vi "Get_Disc_Flow_Rate.vi"(9 "Jet Frequency":dbl, 10 "Radius":dbl[](array[numeric]), 11 "Phase Average":dbl[][](array[numeric])) -> (1 "time":dbl[](array[numeric]), 2 "|Qd|":dbl, 3 "Qd(t)":dbl[](array[numeric]))   [LabVIEW 2012]
uses:
  <vilib>/Analysis/2dsp.llb/Integral Method.ctl
  <vilib>/Analysis/1siggen.llb/Ramp Pattern by Samples.vi
  <vilib>/Analysis/8numeric.llb/1D Numeric Integration.vi
  <vilib>/Analysis/NI_AALBase.lvlib
  <vilib>/gmath/NI_Gmath.lvlib
  <vilib>/Analysis/NI_AALPro.lvlib
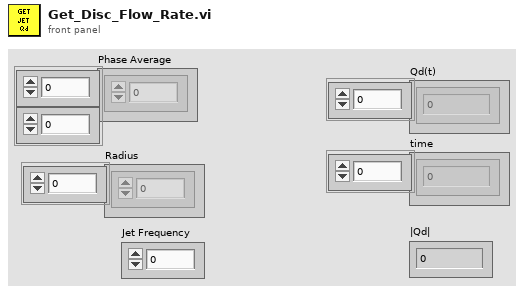
[diagram p1: front panel]
types:
  T1 = typedef "NI_AALPro.lvlib/Integral Method.ctl" = i32
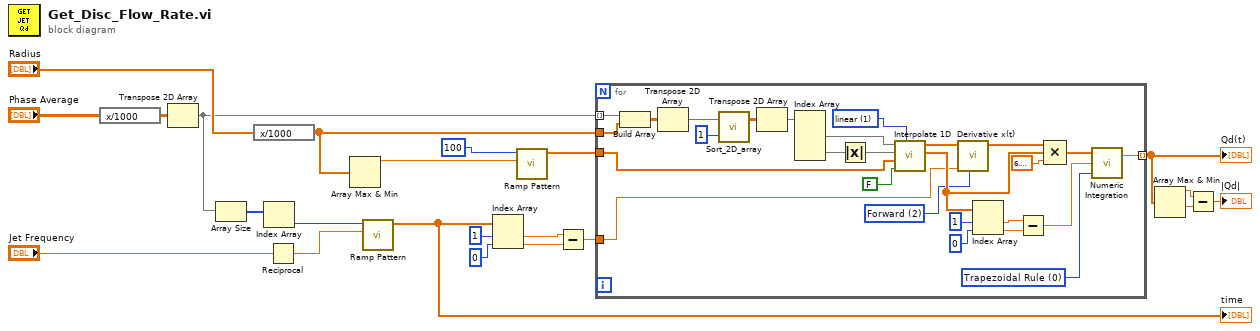
[diagram p0: block diagram]
diagram:
  n1 = expression code="x/1000"("Phase Average") -> (w1:dbl[][])
  n2 = Transpose 2D Array(2D array=w1) -> (transposed array=w16:dbl[][])
  n3 = Array Size(array=w16) -> (size(s)=w15:i32[])
  n4 = expression code="x/1000"("Radius") -> (w3:dbl[])
  n5 = Index Array(array=w15) -> (element=w14:i32)  [unwired: 1 in]
  n6 = Reciprocal(x="Jet Frequency") -> (1/x=w17:dbl)
  n7 = Array Max & Min(array=w3) -> (max value=w20:dbl)  [unwired: 3 out]
  n8 = call-poly <vilib>:"Ramp Pattern.vi"("end"=w17, "samples"=w14) -> ("Ramp Pattern"=w11:dbl[])  [unwired: 8 in, 1 out]
  "time" <- w11
  n9 = Index Array(array=w11, index #1=1 ("index"), index #2=0 ("index")) -> (element #1=w10:dbl, element #2=w9:dbl)
  n10 = call-poly <vilib>:"Ramp Pattern.vi"("end"=w20, "samples"=100) -> ("Ramp Pattern"=w19:dbl[])  [unwired: 8 in, 1 out]
  n11 = Subtract(x=w10, y=w9) -> (x-y=w8:dbl)
  n12 = for {
    tunnel: w3 -> [w43]
    tunnel: w16 -> [w44] mode=indexing
    tunnel: w19 -> [w39]
    tunnel: [w24] -> w7 mode=indexing
    tunnel: w8 -> [w23]
    w38 = 1 items=["nearest", "linear", "spline", "cubic Hermite", "Lagrange"] ("method")
    w27 = u16 2 items=["2nd Order Central", "4th Order Central", "Forward", "Backward"] ("method")
    w31 = T1 0 items=["Trapezoidal Rule", "Simpson's Rule", "Simpson's 3/8 Rule", "Bode Rule"] ("integration method")
    n13 = Build Array(w44, w43) -> (w45:dbl[][])
    n14 = Transpose 2D Array(2D array=w45) -> (transposed array=w47:dbl[][])
    n15 = call "Sort_2D_array.vi"("Column index to sort on"=1, "unsorted array"=w47) -> ("sorted array"=w48:dbl[][])  [unwired: 1 out]
    n16 = Transpose 2D Array(2D array=w48) -> (transposed array=w46:dbl[][])
    n17 = Index Array(array=w46) -> (element #1=w41:dbl[], element #2=w42:dbl[])  [unwired: 4 in]
    n18 = Absolute Value(x=w42) -> (abs(x)=w40:dbl[])
    n19 = call <vilib>:"Interpolate 1D.vi"("method"=w38, "X is monotonic"=FALSE, "xi"=w39, "X"=w40, "Y"=w41) -> ("xi used"=w28:dbl[], "yi"=w26:dbl[])  [unwired: 4 in, 1 out]
    n20 = call <vilib>:"Derivative x(t).vi"("method"=w27, "dt"=w23, "X"=w26) -> ("dX/dt"=w25:dbl[])  [unwired: 7 in, 1 out]
    n21 = Index Array(array=w28, index #1=1 ("index"), index #2=0 ("index")) -> (element #1=w36:dbl, element #2=w35:dbl)
    n22 = Subtract(x=w36, y=w35) -> (x-y=w32:dbl)
    n23 = Compound Arithmetic op=MULTIPLY(w25, w28, 6.283185307179586) -> (w30:dbl[])
    n24 = call-poly <vilib>:"Numeric Integration.vi"("integration method"=w31, "dt"=w32, "Input Array"=w30) -> ("result"=w24:dbl)  [unwired: 1 out]
  }
  "Qd(t)" <- w7
  n25 = Array Max & Min(array=w7) -> (max value=w6:dbl, min value=w5:dbl)  [unwired: 2 out]
  n26 = Subtract(x=w6, y=w5) -> (x-y=→"|Qd|":dbl)
